vi "Receive I32.vi"(8 "error in (no error)":errorcluster, 10 "Broadcast I32 Msg":refnum<class "Broadcast I32 Msg.lvclass">, 11 "TopLevelApplication In":refnum<class "TopLevelApplication.lvclass">) -> (0 "error out":errorcluster, 3 "TopLevelApplication Out":refnum<class "TopLevelApplication.lvclass">)   [LabVIEW 2015, in "TopLevelApplication.lvlib" / "TopLevelApplication.lvclass"]
uses:
  TopLevelApplication.lvclass
  IViewable/IViewable Messages/Broadcast I32 Msg/Broadcast I32 Msg.lvclass
  TopLevelApplication Messages/Test Dialog Return Msg/Test Dialog Return Msg.lvclass
  TopLevelApplication Messages/Test Dialog Return Msg/Test Dialog Return Msg.lvclass/Test Dialog Return Msg.ctl
  IViewable/IViewable Messages/Broadcast I32 Msg/Broadcast I32 Msg.lvclass/Broadcast I32 Msg.ctl
  Dialog Box Implementations/TwoButtonDialogBox/TwoButtonDialogBox.lvclass
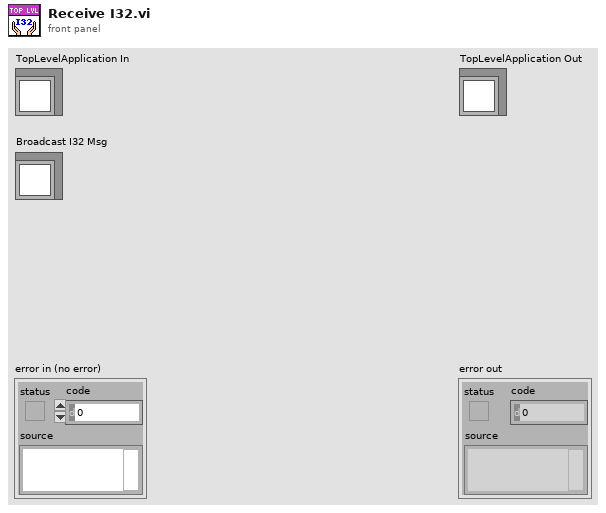
[diagram p1: front panel]
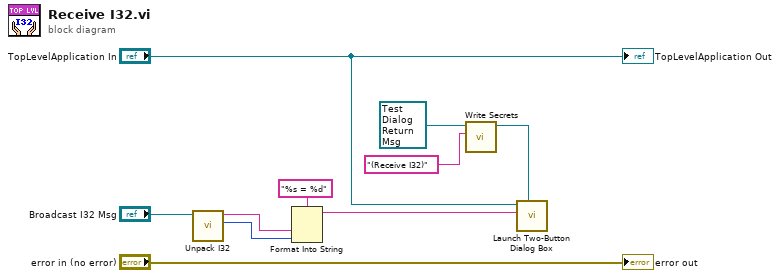
[diagram p0: block diagram]
diagram:
  n1 = call "Unpack I32.vi"("Broadcast I32 Msg In"="Broadcast I32 Msg") -> ("Value"=w8:i32, "Name"=w2:string)  [unwired: 9 in]
  n2 = Format Into String(format string="%s = %d", w2, w8) -> (resulting string=w5:string)  [unwired: 2 in, 1 out]
  n3 = call "Write Secrets.vi"("Secrets"="(Receive I32)", "Test Dialog Return Msg in"=refnum<class "Test Dialog Return Msg.lvclass"> refnum ("TopLevelApplication.lvlib:Test Dialog Return Msg.lvclass")) -> ("Test Dialog Return Msg out"=w3:refnum<class "Test Dialog Return Msg.lvclass">)  [unwired: 8 in, 1 out]
  n4 = call "Launch Two-Button Dialog Box.vi"("True Button Return Message (Optional)"=w3, "Message Text"=w5, "Dialog Launcher"="TopLevelApplication In") -> ()  [unwired: 8 in, 1 out]
  "error out" <- "error in (no error)"
  "TopLevelApplication Out" <- "TopLevelApplication In"
